vi "Disable Debugging.vi"(8 "error in (no error)":errorcluster, 11 "VI Reference In":refnum<vi>) -> (0 "error out":errorcluster, 3 "VI Reference Out":refnum<vi>)   [LabVIEW 2015]
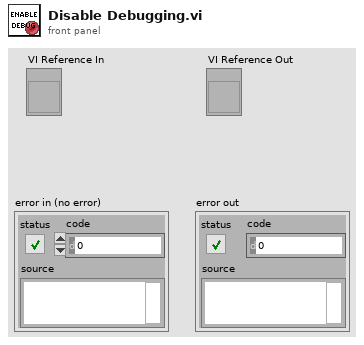
[diagram p1: front panel]
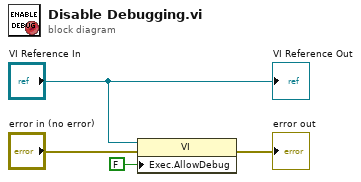
[diagram p0: block diagram]
diagram:
  n1 = property class="VI"(reference="VI Reference In", error in="error in (no error)", "Exec.AllowDebug"=FALSE ("Execution:Allow Debugging")) -> (error out=→"error out":errorcluster)  [unwired: 1 out]
  "VI Reference Out" <- "VI Reference In"
